vi "Begin.vi"(8 "error in (no error)":errorcluster, 9 "Reverse solenoid channel":T1, 10 "Forward Solenoid Channel":T1, 11 "Solenoids in":refnum<class "Solenoids.lvclass">) -> (0 "error out":errorcluster, 3 "Solenoids out":refnum<class "Solenoids.lvclass">)   [LabVIEW 2018, in "Pneumatics control.lvlib" / "Solenoids.lvclass"]
doc: "Opens a solenoid channel."
uses:
  Solenoids.lvclass
  <vilib>/Rock Robotics/WPI/Solenoid/WPI_SolenoidChannel.ctl
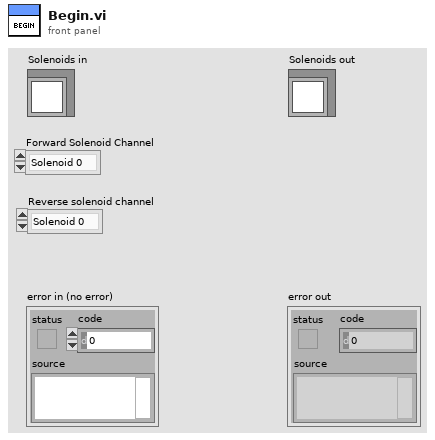
[diagram p1: front panel]
types:
  T1 = typedef "WPI_SolenoidChannel.ctl" = enum8{"Solenoid 0", "Solenoid 1", "Solenoid 2", "Solenoid 3", "Solenoid 4", "Solenoid 5", "Solenoid 6", "Solenoid 7", "Invalid"}
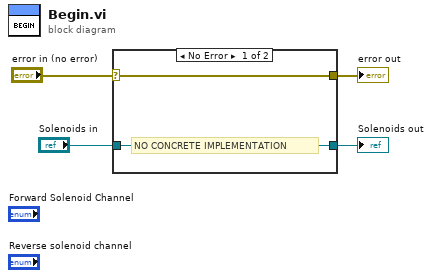
[diagram p0: block diagram]
diagram:
  n1 = case shown="No Error" "error in (no error)" {
    selector: "error in (no error)" -> [w5 w8]
    tunnel: [w5 w8] -> w3
    tunnel: [w6 w7] -> w1
    tunnel: "Solenoids in" -> [w6 w7]
    frame No Error {
      # "NO CONCRETE IMPLEMENTATION"
    }
    frame Error {
    }
  }
  "error out" <- w3
  "Solenoids out" <- w1
